vi "CurrentTime(H).vi"(8 "error in (no error)":errorcluster) -> (0 "error out":errorcluster, 1 "Current Time (Hours)":dbl)   [LabVIEW 2009]
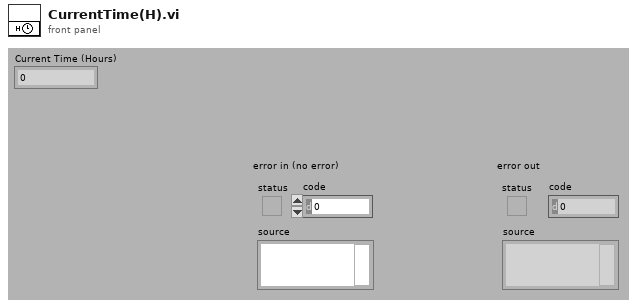
[diagram p1: front panel]
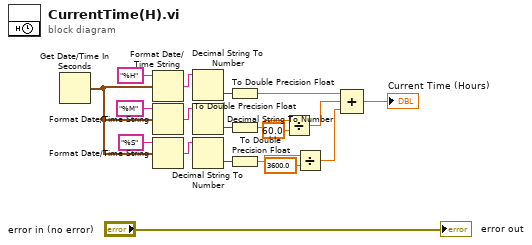
[diagram p0: block diagram]
diagram:
  n1 = Get Date/Time In Seconds() -> (seconds since 1Jan1904=w2:timestamp)
  n2 = Format Date/Time String(time format string (%c)="%H", seconds (now)=w2) -> (date/time string=w15:string)  [unwired: 1 out]
  n3 = Format Date/Time String(time format string (%c)="%M", seconds (now)=w2) -> (date/time string=w14:string)  [unwired: 1 out]
  n4 = Format Date/Time String(time format string (%c)="%S", seconds (now)=w2) -> (date/time string=w8:string)  [unwired: 1 out]
  n5 = Decimal String To Number(string=w15) -> (number=w19:i32)  [unwired: 3 out]
  n6 = Decimal String To Number(string=w14) -> (number=w16:i32)  [unwired: 3 out]
  n7 = Decimal String To Number(string=w8) -> (number=w6:i32)  [unwired: 3 out]
  n8 = To Double Precision Float(number=w19) -> (double precision float=w10:dbl)
  n9 = To Double Precision Float(number=w16) -> (double precision float=w13:dbl)
  n10 = To Double Precision Float(number=w6) -> (double precision float=w4:dbl)
  n11 = Divide(x=w13, y=60.0) -> (x/y=w11:dbl)
  n12 = Divide(x=w4, y=3600.0) -> (x/y=w3:dbl)
  n13 = Compound Arithmetic op=ADD(w10, w11, w3) -> (→"Current Time (Hours)":dbl)
  "error out" <- "error in (no error)"
